vi "Create Column Definitions.vi"(8 "error in (no error)":errorcluster, 10 "Columns":T1 {"MinWidth" min=2 step=1; "AutoSizeMode" items=["None"=1, "ColumnHeader"=2, "AllCellsExceptHeader"=4, "AllCells"=6, "DisplayedCellsExceptHeader"=8, "DisplayedCells"=10, "Fill"=16]; "FillWeight" min=1 max=100}) -> (0 "error out":errorcluster, 3 "GridColumn out":refnum<class "GridColumn.lvclass">)   [LabVIEW 2014, in "GridColumn.lvclass"]
uses:
  GridColumn.lvclass
  ColumnDefinition.ctl
  GridColumn.lvclass/GridColumn.ctl
  Write Name.vi
  Write datatype.vi
  Write Params.vi
  Write AutoSizeMode.vi
  Write FillWeight.vi
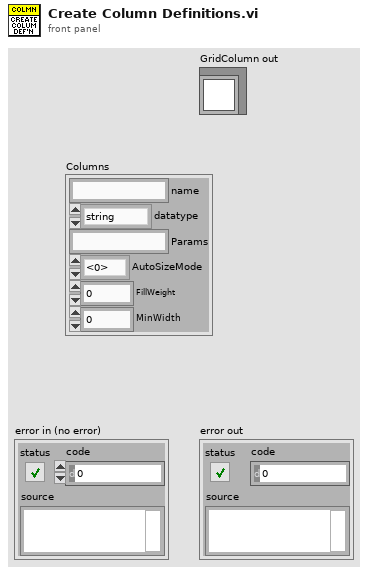
[diagram p1: front panel]
types:
  T1 = typedef "GridColumn.lvclass/ColumnDefinition.ctl" = cluster{"name":string, "datatype":enum16{"string", "image", "check", "numeric", "timestamp", "button", "combo"}, "Params":string, "AutoSizeMode":i32, "FillWeight":sgl, "MinWidth":i32}
  T2 = enum16{"string", "image", "check", "numeric", "timestamp", "button", "combo"}
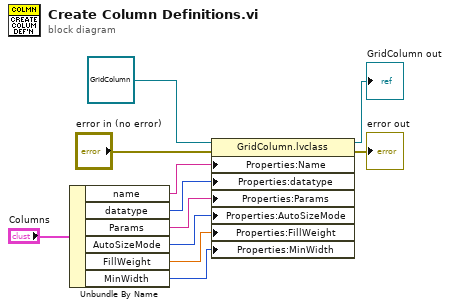
[diagram p0: block diagram]
diagram:
  n1 = Unbundle By Name("Columns") -> ("name"=w8:string, "datatype"=w3:T2, "Params"=w9:string, "AutoSizeMode"=w10:i32, "FillWeight"=w11:sgl, "MinWidth"=w2:i32)
  n2 = property class="GridColumn.lvclass"(reference=refnum<class "GridColumn.lvclass"> refnum ("GridColumn in"), error in="error in (no error)", "Properties:Name"=w8, "Properties:datatype"=w3, "Properties:Params"=w9, "Properties:AutoSizeMode"=w10, "Properties:FillWeight"=w11, "Properties:MinWidth"=w2) -> (reference out=→"GridColumn out":refnum<class "GridColumn.lvclass">, error out=→"error out":errorcluster)
